vi "oscilloscope.vi"() -> ()   [LabVIEW 2013]
uses:
  <instrlib>/Tektronix TDS 200 1000 2000 Series/Tektronix TDS 200 1000 2000 Series.lvlib
panel:
  out "x < y?":bool
  out "Y":dbl
  in  "stop":bool
  out "Waveform Data":waveform(dbl)(graph)
  in  "Source (0: Channel 1)":u16(ring) items=["Channel 1", "Channel 2", "Channel 3", "Channel 4", "Math", "Reference A", "Reference B", "Reference C", "Reference D", "FFT"]
  in  "Serial Configuration":T1={"Baud Rate"=9600, "Parity"=0, "Stop Bits"=10, "Flow Control"=2} {"Flow Control" items=["None", "XON/XOFF", "RTS/CTS", "XON/XOFF & RTS/CTS", "DTR/DSR", "XON/XOFF & DTR/DSR"]; "Stop Bits" items=["1.0"=10, "1.5"=15, "2.0"=20]; "Parity" items=["None", "Odd", "Even", "Mark", "Space"]; "Baud Rate" items=["300"=300, "600"=600, "1200"=1200, "2400"=2400, "4800"=4800, "9600"=9600, "19200"=19200]}
  in  "VISA resource name":refnum<visa-resource-name>
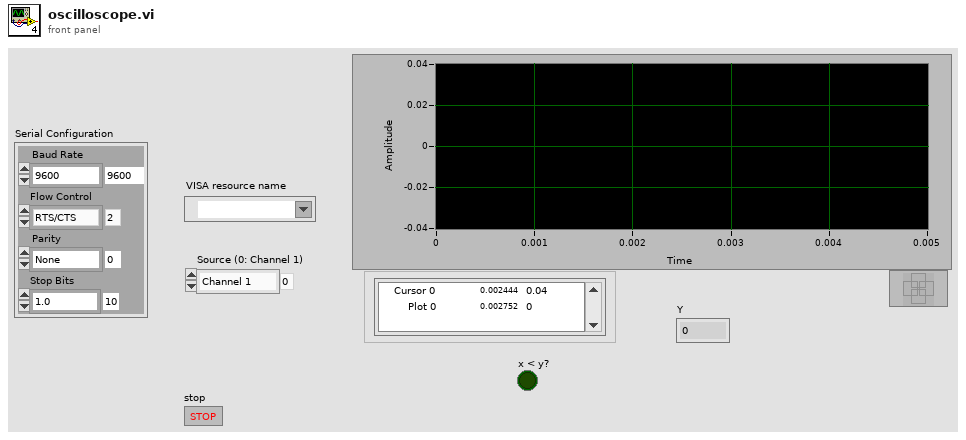
[diagram p1: front panel]
types:
  T1 = cluster{"Baud Rate":u32, "Parity":u16, "Stop Bits":u16, "Flow Control":u16}
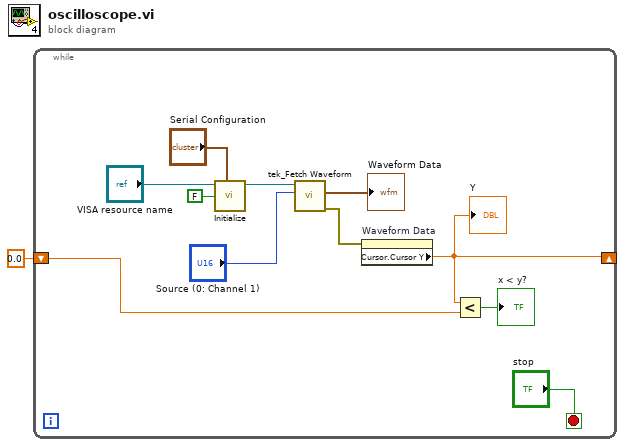
[diagram p0: block diagram]
diagram:
  n1 = while {
    shift-right: [w4] -> _
    shift-left: 0.0 ("Cursor.Cursor Y") -> [w3]
    stop <- "stop" stop-if-true
    n2 = call <instrlib>:"Initialize.vi"("Serial Configuration"="Serial Configuration", "Reset? (T: Yes)"=FALSE, "VISA resource name"="VISA resource name") -> ("VISA resource name out"=w9:refnum<visa-resource-name>)  [unwired: 7 in, 1 out]
    n3 = call "tek_Fetch Waveform.vi"("Source (0: Channel 1)"="Source (0: Channel 1)", "VISA resource name"=w9) -> ("error out"=w5:errorcluster, "Waveform Data"=→"Waveform Data":waveform(dbl))  [unwired: 4 in, 4 out]
    n4 = property on="Waveform Data" class="WFGraph (strict)"(error in=w5) -> ("Cursor.Cursor Y"=w4:dbl)  [unwired: 1 in, 2 out]
    "Y" <- w4
    n5 = Less?(x=w4, y=w3) -> (x < y?=→"x < y?":bool)
  }
